vi "Demande saisie OF.vi"(8 "entrée d'erreur (pas d'erreur)":errorcluster, 10 "Part Number PCBA":string(combo), 11 "Type Product":string(combo)) -> (0 "sortie d'erreur":errorcluster, 3 "Continuer":bool)   [LabVIEW 2020]
uses:
  Class/Test/Enter_Batch/Enter_Batch.lvclass
  C:/Users/ngarcin/OneDrive - Altyor/Standard TB/Class/Test/Test (Default)/Test (Default).lvclass
  <vilib>/Utility/config.llb/Read Key (String).vi
  Commun VI/Library Commun.lvlib
  <vilib>/Utility/config.llb/NI_LVConfig.lvlib
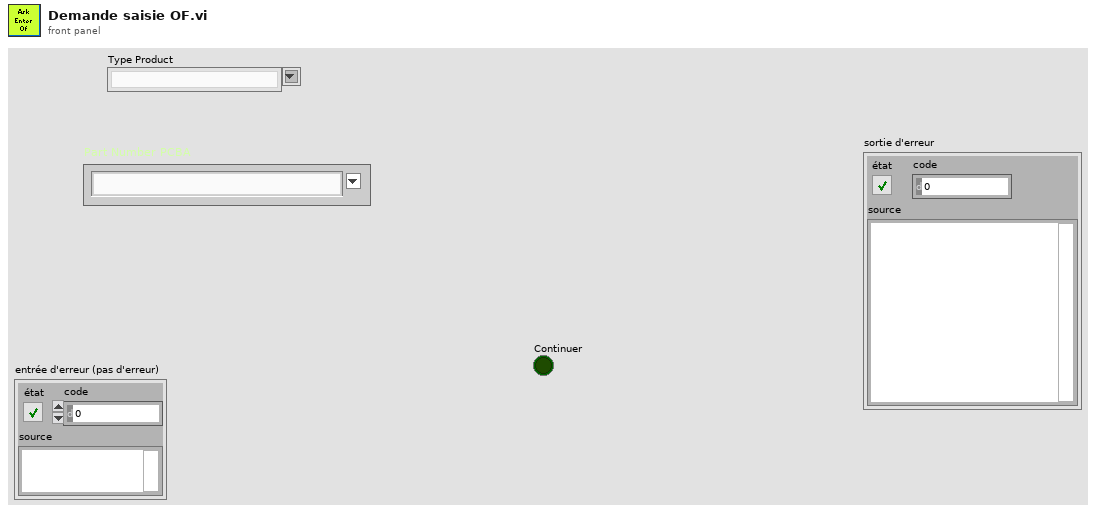
[diagram p1: front panel]
types:
  T1 = typedef "NI_LVConfig.lvlib/Config Data RefNum.ctl" = refnum<k1>
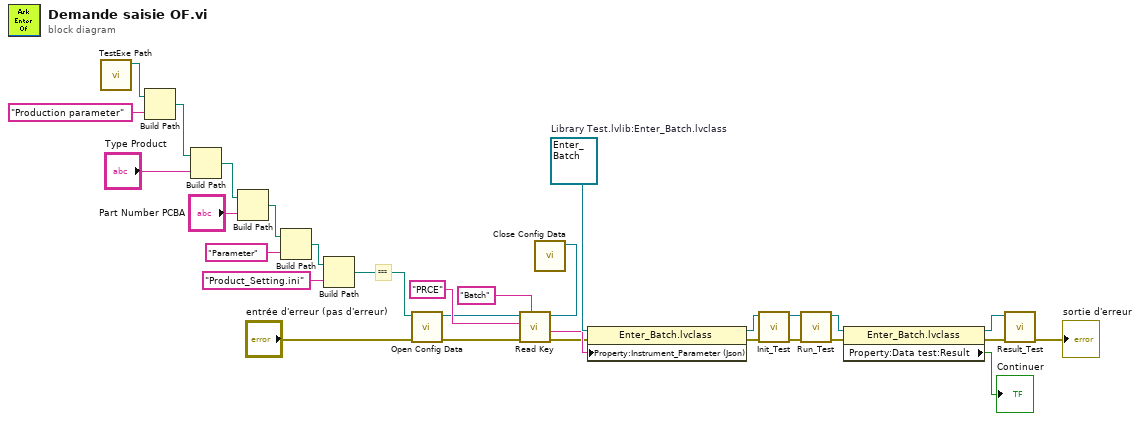
[diagram p0: block diagram]
diagram:
  w22 = refnum<class "Enter_Batch.lvclass"> refnum  # Library Test.lvlib:Enter_Batch.lvclass
  # "²²²"
  n1 = call "TestExe Path.vi"() -> ("Chemin Actuel"=w17:path)  [unwired: 9 in, 2 out]
  n2 = Build Path(base path=w17, name or relative path="Production parameter" ("nom ou chemin relatif")) -> (appended path=w16:path)
  n3 = Build Path(base path=w16, name or relative path="Type Product") -> (appended path=w15:path)
  n4 = Build Path(base path=w15, name or relative path="Part Number PCBA") -> (appended path=w14:path)
  n5 = Build Path(base path=w14, name or relative path="Parameter" ("nom ou chemin relatif")) -> (appended path=w12:path)
  n6 = Build Path(base path=w12, name or relative path="Product_Setting.ini" ("nom ou chemin relatif")) -> (appended path=w7:path)
  n7 = call <vilib>:"Open Config Data.vi"("error in (no error)"="entrée d'erreur (pas d'erreur)", "configuration file path"=w7) -> ("error out"=w5:errorcluster, "refnum"=w1:T1)  [unwired: 7 in, 1 out]
  n8 = call-poly <vilib>:"Read Key.vi"("section"="Batch" ("nom ou chemin relatif"), "error in (no error)"=w5, "key"="PRCE", "refnum"=w1) -> ("error out"=w3:errorcluster, "value"=w4:string, "refnum out"=w6:T1)  [unwired: 4 in, 1 out]
  n9 = call <vilib>:"Close Config Data.vi"("refnum"=w6) -> ()  [unwired: 9 in, 2 out]
  n10 = property class="Enter_Batch.lvclass"(reference=w22, error in=w3, "Property:Instrument_Parameter (Json)"=w4) -> (reference out=w21:refnum<class "Enter_Batch.lvclass">, error out=w20:errorcluster)
  n11 = call-dynamic "Init_Test.vi"("error in (no error)"=w20, "Delay en entrée"=w21) -> ("error out"=w29:errorcluster, "Delay en sortie"=w30:refnum<class "Enter_Batch.lvclass">)  [unwired: 8 in]
  n12 = call-dynamic "Run_Test.vi"("error in (no error)"=w29, "Test (Default) en entrée"=w30) -> ("error out"=w25:errorcluster, "Test (Default) en sortie"=w24:refnum<class "Enter_Batch.lvclass">)  [unwired: 8 in]
  n13 = property class="Enter_Batch.lvclass"(reference=w24, error in=w25) -> (reference out=w28:refnum<class "Enter_Batch.lvclass">, error out=w26:errorcluster, "Property:Data test:Result"=→"Continuer":bool)
  n14 = call-dynamic "Result_Test.vi"("error in (no error)"=w26, "Delay en entrée"=w28) -> ("error out"=→"sortie d'erreur":errorcluster)  [unwired: 8 in, 1 out]
